vi "h.ACQ.ParsePeaksData.vi"(1 "Data from #GetPeaks":u8[](array[numeric])) -> (0 "Peaks Data":T1 {"Peaks Wvls, nm"."Peak Wvls, nm" format="%#_8g"})   [LabVIEW 2019, in "h.Library.lvlib"]
doc: "This vi parses the data from the h.DAQ.GetPeaks.vi and returns a PeaksData cluster that contains the transfered peaks data.\n\n<b>Data from #GetPeaks</b> - The data returned by the #GetPeaks command\n<b>Peaks Data</b> - cluster containing the peaks data and supporting information"
uses:
  h.Library.lvlib
  CTL/h.ACQ.PeaksData.ctl
  CTL/h.ACQ.PeaksWvl.ctl
panel:
  # "Hyperion Parse #GetPeaks Data"
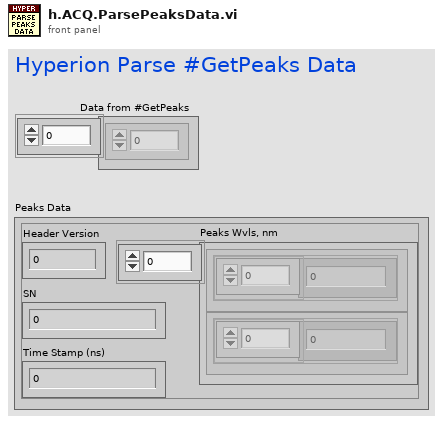
[diagram p1: front panel]
types:
  T1 = typedef "h.Library.lvlib/h.ACQ.PeaksData.ctl" = cluster{"SN":u64, "Time Stamp (ns)":u64, "Header Version":u16, "Peaks Wvls, nm":T2[]}
  T2 = typedef "h.Library.lvlib/h.ACQ.PeaksWvl.ctl" = cluster{"Peak Wvls, nm":dbl[]}
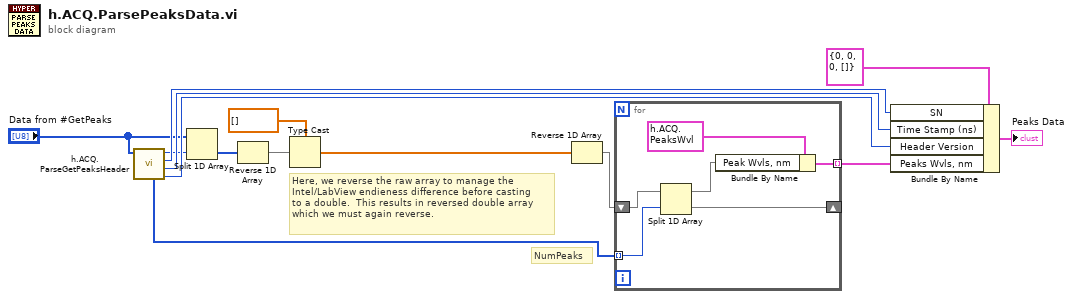
[diagram p0: block diagram]
diagram:
  # "NumPeaks"
  # "Here, we reverse the raw array to manage the\nIntel/LabView endieness difference before casting\nto a double.  This results in reversed double array\nwhich we must again reverse."
  n1 = call "h.ACQ.ParseGetPeaksHeader.vi"("Header from #GetPeaks"="Data from #GetPeaks") -> ("Header Version"=w14:u16, "Time Stamp (ns)"=w13:u64, "SN"=w12:u64, "Header Length"=w8:u16, "#Peaks"=w6:u16[])  [unwired: 6 in]
  n2 = Split 1D Array(array="Data from #GetPeaks", index=w8) -> (second subarray=w2:u8[])  [unwired: 1 out]
  n3 = Reverse 1D Array(array=w2) -> (reversed array=w4:u8[])
  n4 = Type Cast(type=dbl[] [], x=w4) -> (*(type *) &x=w3:dbl[])
  n5 = Reverse 1D Array(array=w3) -> (reversed array=w7:dbl[])
  n6 = for {
    tunnel: w6 -> [w19] mode=indexing
    shift-right: [w18] -> _
    shift-left: w7 -> [w20]
    tunnel: [w16] -> w11 mode=indexing
    n7 = Split 1D Array(array=w20, index=w19) -> (first subarray=w17:dbl[], second subarray=w18:dbl[])
    n8 = Bundle By Name(cluster=T2 {"Peak Wvls, nm"=[1512.9051860814243, 1515.5702637018003, 1519.0474862664064, 1521.9970748811888, 1524.5764290572702, 1528.159016640387, 1530.475549907591, 1534.1043393370621, 1537.4124500994837, 1539.8441852982514, 1542.9230343767763, 1545.8173501630033, 1549.0146817641494, 1551.8023413606945, 1554.5670023154048, 1559.1001620675313, 1561.538122059349, 1564.474074928091, 1566.2899965170764, 1569.9593940437987, 1573.222828330526, 1575.9746411171434, 1578.8718374756434, 1581.827770883752, 1584.3136832174469]} ("Ch"), "Peak Wvls, nm"=w17) -> (w16:T2)
  }
  n9 = Bundle By Name(cluster=T1 {"SN"=0, "Time Stamp (ns)"=0, "Header Version"=0, "Peaks Wvls, nm"=[]} ("Peaks Data"), "SN"=w12, "Time Stamp (ns)"=w13, "Header Version"=w14, "Peaks Wvls, nm"=w11) -> (→"Peaks Data":T1)
